vi "pid_test_heat_temp.vi"() -> ()   [LabVIEW 2019]
uses:
  <vilib>/addons/control/pid/pid.llb/PID (DBL).vi
  <vilib>/addons/control/pid/NI_PID_pid.lvlib
panel:
  out "Temp Diff":cluster{dbl[], dbl[]}(graph)
  out "Volt Diff":cluster{dbl[], dbl[]}(graph)
  out "Temp":cluster{dbl[], dbl[]}[](graph)
  out "Volt":cluster{dbl[], dbl[]}(graph)
  in  "sample_mass":dbl
  in  "sample_heat_cap":dbl
  in  "heater_res":dbl
  in  "ambient_temp":dbl
  in  "sample_temp":dbl
  in  "dt":dbl
  in  "stop":bool
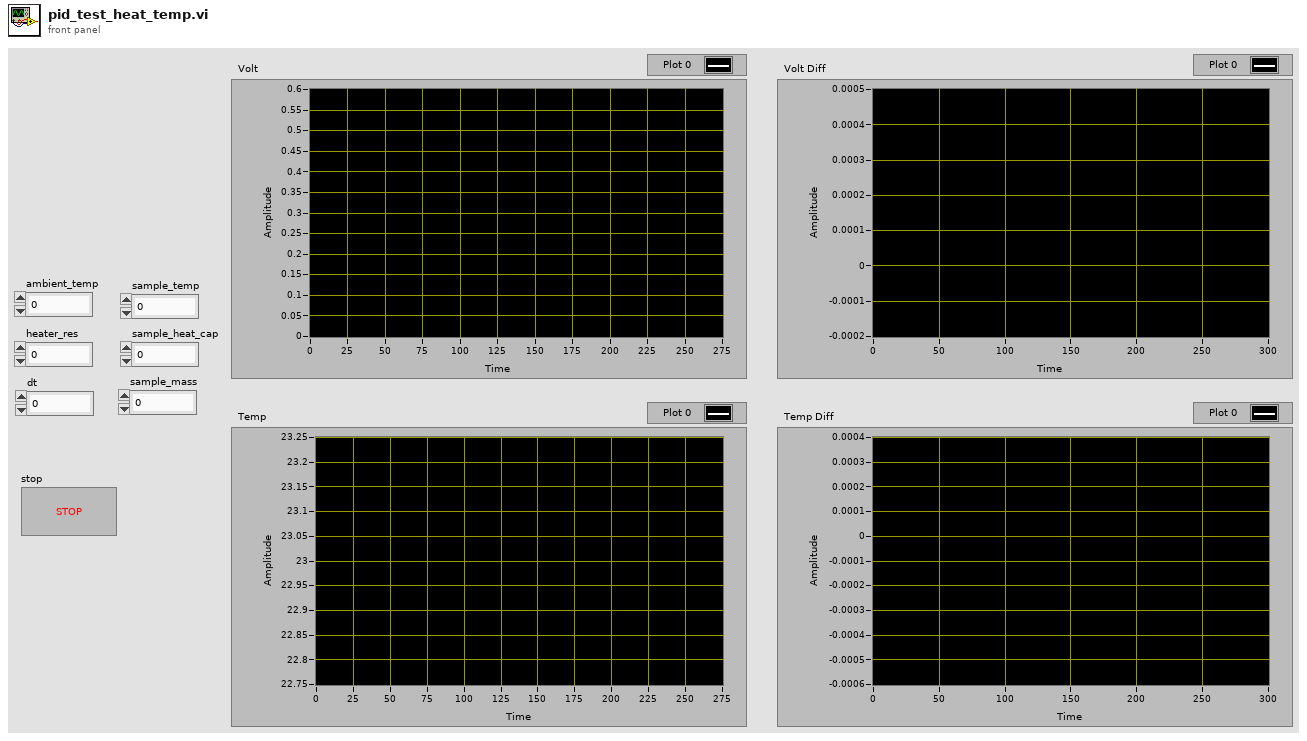
[diagram p1: front panel]
types:
  T1 = cluster{"proportional gain (Kc)":dbl, "integral time (Ti, min)":dbl, "derivative time (Td, min)":dbl}
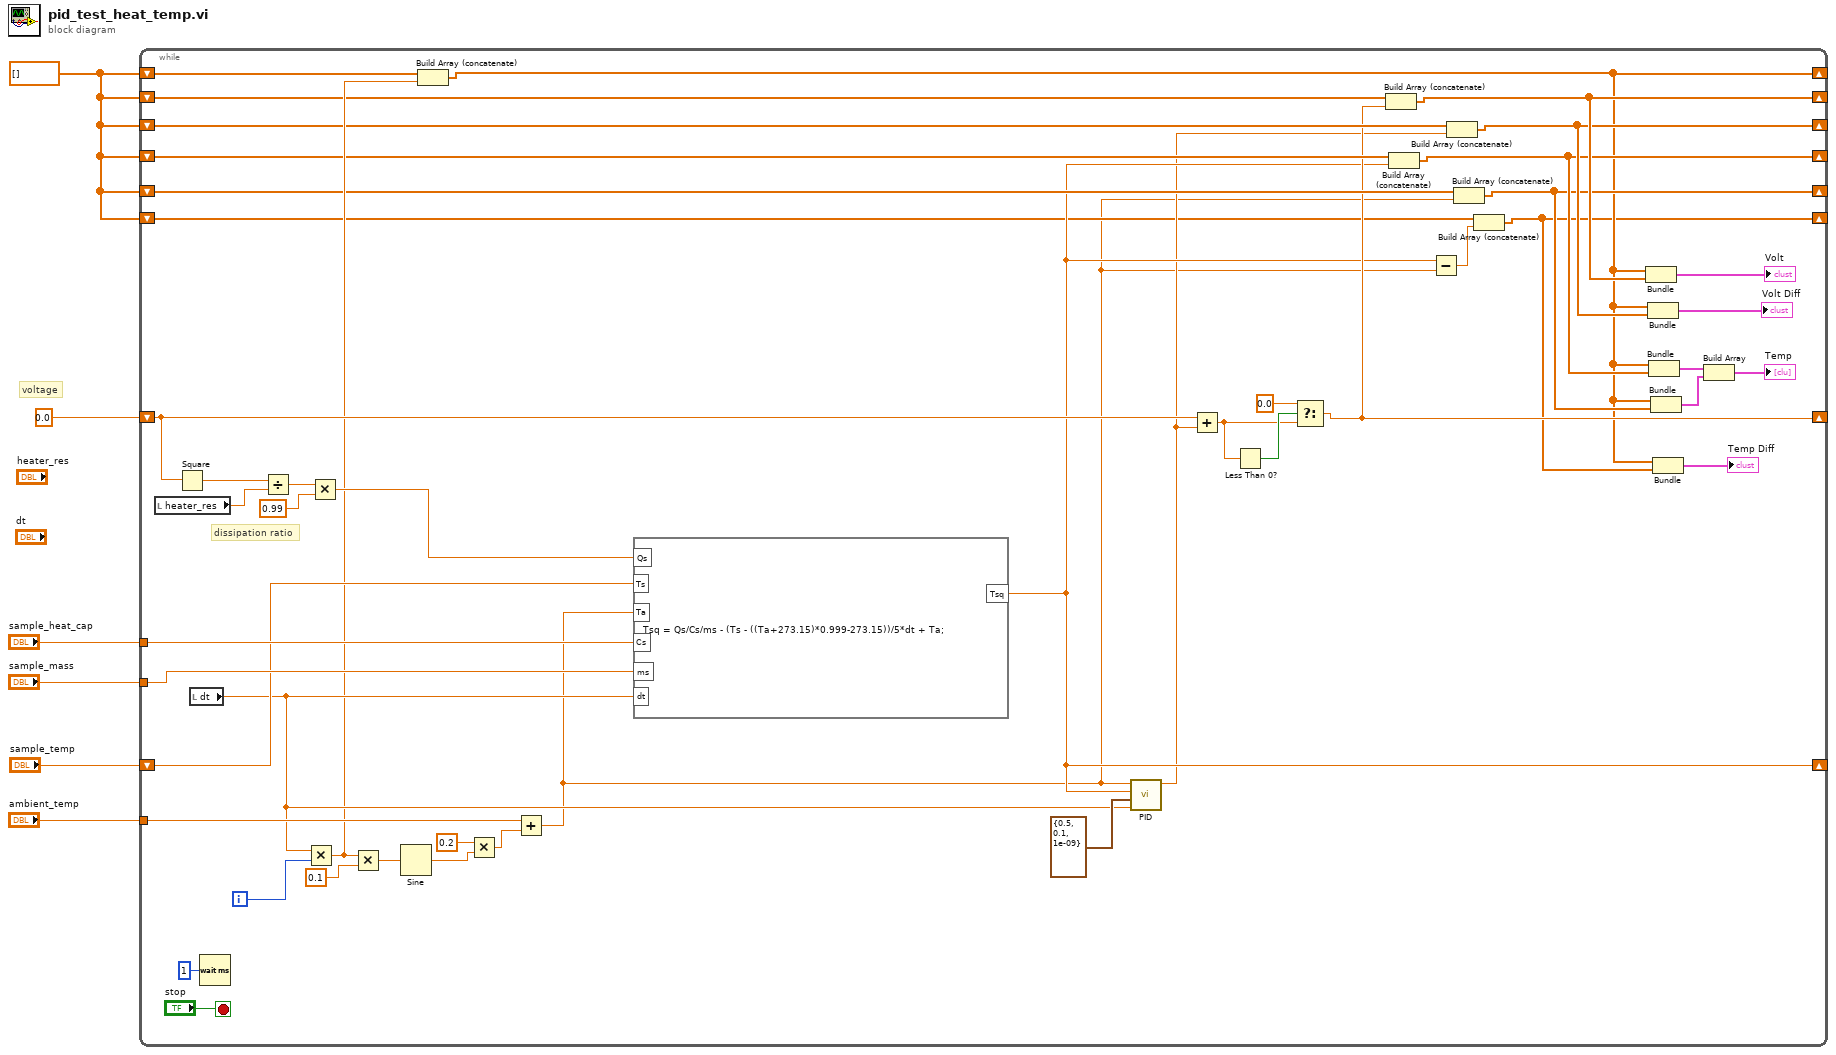
[diagram p0: block diagram]
diagram:
  w1 = dbl[] []
  # "voltage"
  n1 = while {
    shift-right: [w10] -> _
    shift-left: w1 -> [w33]
    shift-right: [w17] -> _
    shift-left: 0.0 -> [w34]
    tunnel: "sample_heat_cap" -> [w46]
    tunnel: "sample_mass" -> [w45]
    shift-right: [w14] -> _
    shift-left: "sample_temp" -> [w37]
    tunnel: "ambient_temp" -> [w38]
    shift-right: [w27] -> _
    shift-left: w1 -> [w31]
    shift-right: [w23] -> _
    shift-left: w1 -> [w30]
    shift-right: [w26] -> _
    shift-left: w1 -> [w29]
    shift-right: [w22] -> _
    shift-left: w1 -> [w28]
    shift-right: [w8] -> _
    shift-left: w1 -> [w12]
    i -> [w44]
    stop <- "stop" stop-if-true
    # "dissipation ratio"
    n2 = local read "heater_res"() -> (w50:dbl)
    n3 = Square(x=w34) -> (x^2=w51:dbl)
    n4 = local read "dt"() -> (w35:dbl)
    n5 = Wait (ms)(milliseconds to wait=u32 1) -> ()  [unwired: 1 out]
    n6 = Divide(x=w51, y=w50) -> (x/y=w49:dbl)
    n7 = Multiply(x=w35, y=w44) -> (x*y=w32:dbl)
    n8 = Multiply(x=w49, y=0.99) -> (x*y=w47:dbl)
    n9 = Multiply(x=w32, y=0.1) -> (x*y=w42:dbl)
    n10 = Sine(x=w42) -> (sin(x)=w41:dbl)
    n11 = Build Array (concatenate)(w33, w32) -> (w10:dbl[])
    n12 = Multiply(x=0.2, y=w41) -> (x*y=w39:dbl)
    n13 = Add(x=w38, y=w39) -> (x+y=w7:dbl)
    n14 = formula code="Tsq = Qs/Cs/ms - (Ts - ((Ta+273.15)*0.999-273.15))/5*dt + Ta;"("Ts"=w37, "Qs"=w47, "Ta"=w7, "Cs"=w46, "ms"=w45, "dt"=w35) -> ("Tsq"=w14:dbl)
    n15 = call-poly <vilib>:"PID.vi"("dt (s)"=w35, "PID gains"=T1 {"proportional gain (Kc)"=0.5, "integral time (Ti, min)"=0.1, "derivative time (Td, min)"=1e-09}, "process variable"=w14, "setpoint"=w7) -> ("output"=w13:dbl)  [unwired: 6 in, 1 out]
    n16 = Add(x=w34, y=w13) -> (x+y=w18:dbl)
    n17 = Less Than 0?(x=w18) -> (x < 0?=w20:bool)
    n18 = Select(t=0.0, s=w20, f=w18) -> (s? t:f=w17:dbl)
    n19 = Build Array (concatenate)(w31, w17) -> (w27:dbl[])
    n20 = Build Array (concatenate)(w30, w14) -> (w23:dbl[])
    n21 = Subtract(x=w14, y=w7) -> (x-y=w11:dbl)
    n22 = Build Array (concatenate)(w29, w13) -> (w26:dbl[])
    n23 = Build Array (concatenate)(w28, w7) -> (w22:dbl[])
    n24 = Build Array (concatenate)(w12, w11) -> (w8:dbl[])
    n25 = Bundle(w10, w27) -> (→"Volt":cluster{dbl[], dbl[]})  [unwired: 1 in]
    n26 = Bundle(w10, w26) -> (→"Volt Diff":cluster{dbl[], dbl[]})  [unwired: 1 in]
    n27 = Bundle(w10, w23) -> (w24:cluster{dbl[], dbl[]})  [unwired: 1 in]
    n28 = Bundle(w10, w22) -> (w25:cluster{dbl[], dbl[]})  [unwired: 1 in]
    n29 = Bundle(w10, w8) -> (→"Temp Diff":cluster{dbl[], dbl[]})  [unwired: 1 in]
    n30 = Build Array(w24, w25) -> (→"Temp":cluster{dbl[], dbl[]}[])
  }
